vi "Relay Data Stream Control (Slow side, Output).vi"(4 "ready for input?":bool=TRUE caption="ready for input? (true)", 5 "state handshake":T1, 6 "force error":bool caption="force error (false)", 7 "stream.num samples 0":u64, 9 "data valid":bool=TRUE caption="data valid (true)", 10 "element count":u16=1 caption="element count (1)", 11 "stream.request state 0":T2) -> (0 "request data":bool, 1 "send data":bool, 2 "stream.state 0":T2, 3 "stream.metadata 0":u64)   [LabVIEW 2014, in "niInstr Streaming v1 FPGA.lvlib"]
doc: "<B>General</B>\n\nThis VI gates the assertion of <B>Send Data?</B> with a state machine controller. This enables the control and monitoring of finite and continuous streams of data.\n\n<B>Signals</B>\n\nThe stream is controlled by the <B>stream.request state</B> and <B>stream.num samples</B> inputs. The stream is monitored by the <B>stream.state</B> and <B>stream.samples transferred</B> outputs.\n\nWhen <B>Data Valid</B> is True, and <B>Ready for Input?</B> is True, the state machine will assert <B>Send Data?</B> until the transfer completes.\n\nWhen <B>Data Valid</B> is True, but <B>Ready for Input?</B> is False, the stream stops asserting <B>Send Data</B> and enters the \"Overflow\" state.\n\nWhen <B>Force Error</B> is True, the stream is forced into the Overflow state. This allows user logic to monitor for fatal conditions and stop the stream.\n\n<B>Operation</B>\n\nThe state machine has two fundamental modes of transfer: \"Finite\" and \"Continuous.\"\n\nIn Finite mode, the state machine will count <B>stream.num samples</B> in increments of <B>Element Count</B>. When the count is equal to or exceeds <B>stream.num samples</B>, it prevents the assertion of <B>Send Data?</B> and enters the Done state. In the \"Done\" state the samples transferred continues to be reported until the user requests that the state machine return to \"Idle.\"\n\nIn Continuous mode, the state machine will behave identically to Finite mode, but will continously transfer samples instead of counting them."
uses:
  <instrlib>/_niInstr/Streaming/v1/FPGA/niInstr Streaming v1 FPGA.lvlib
  <instrlib>/_niInstr/Streaming/v1/Common/Stream State.ctl
  <instrlib>/_niInstr/Streaming/v1/FPGA/Public/Stream Additive Count Register.ctl
  <instrlib>/_niInstr/Streaming/v1/Common/niInstr Streaming v1 Common.lvlib
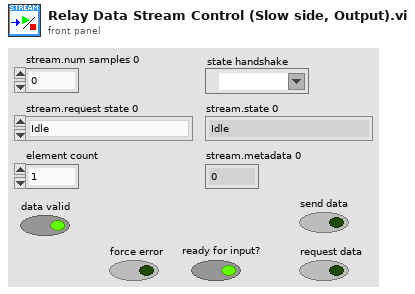
[diagram p1: front panel]
types:
  T1 = typedef "niInstr Streaming v1 FPGA.lvlib/Stream Additive Count Register.ctl" = refnum<k21>
  T2 = typedef "niInstr Streaming v1 Common.lvlib/Stream State.ctl" = enum8{"Idle", "Finite Transfer", "Continuous", "Done", "Overflow", "Not Ready", "Cancel"}
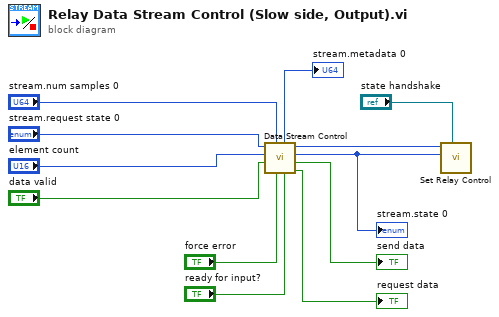
[diagram p0: block diagram]
diagram:
  n1 = call <instrlib>:"Data Stream Control.vi"("ready for input?"="ready for input?", "force error"="force error", "stream.num samples 0"="stream.num samples 0", "data valid"="data valid", "element count"="element count", "stream.request state 0"="stream.request state 0") -> ("request data"=→"request data":bool, "send data"=→"send data":bool, "stream.state 0"=w1:T2, "stream.samples transferred 0"=w12:u64, "stream.metadata 0"=→"stream.metadata 0":u64)  [unwired: 1 in]
  "stream.state 0" <- w1
  n2 = call <instrlib>:"Set Relay Control.vi"("state handshake"="state handshake", "stream.state"=w1, "samples transferred"=w12) -> ()  [unwired: 8 in, 1 out]
